vi "Control iteration 0.vi"(4 "Angle theta [degrees]":dbl, 6 "Number of steps":dbl, 7 "Sweep plane & fixed axis":string, 9 "Current iteration":i32, 10 "Magnetic field strength [µT]":dbl, 11 "Octant":string) -> (0 "Magnetic field z [µT]":dbl, 1 "Magnetic field y [µT]":dbl, 2 "Magnetic field x [µT]":dbl, 3 "Current angle":dbl, 5 "Output instructions iteration 0":string)   [LabVIEW 2018]
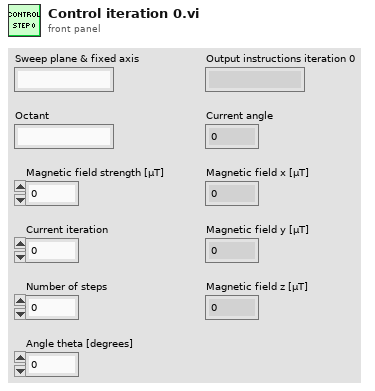
[diagram p1: front panel]
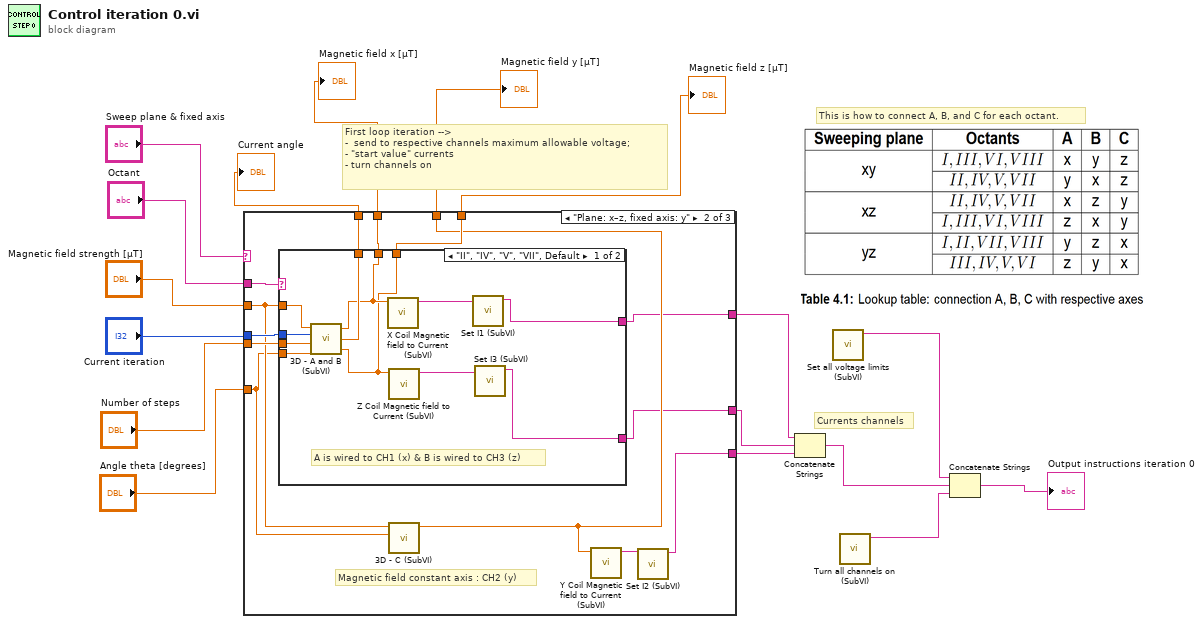
[diagram p0: block diagram]
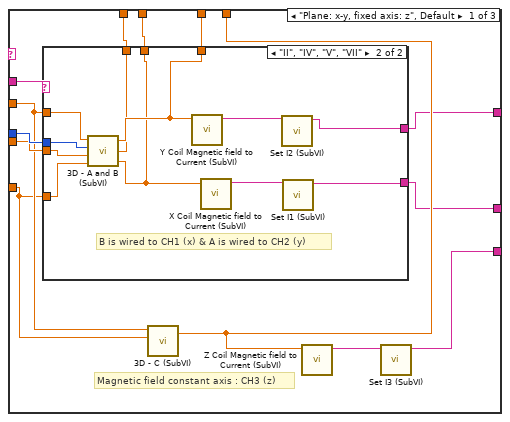
[diagram p2: hidden frame]
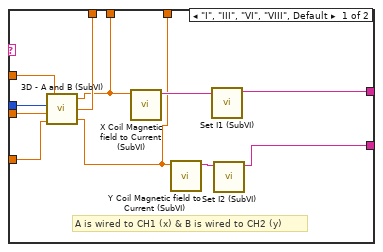
[diagram p3: hidden frame]
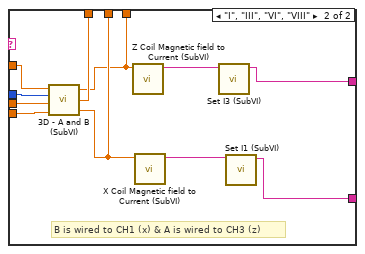
[diagram p4: hidden frame]
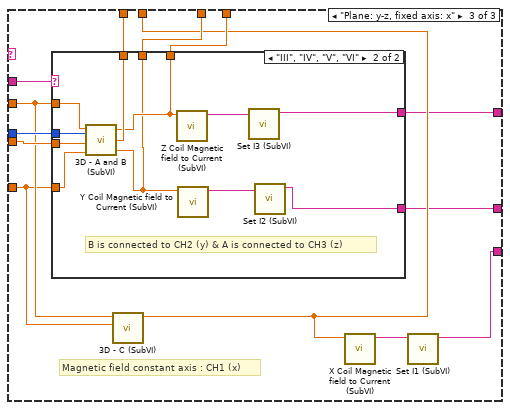
[diagram p5: hidden frame]
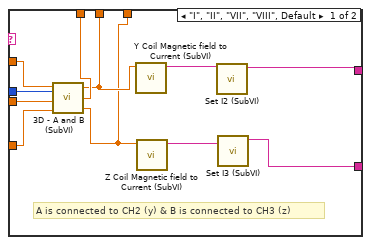
[diagram p6: hidden frame]
diagram:
  # "This is how to connect A, B, and C for each octant."
  # "Currents channels"
  # "First loop iteration -->\n-  send to respective channels maximum allowable voltage;\n- \"start value\" currents\n- turn channels on"
  n1 = case shown="\"Plane: x–z, fixed axis: y\"" "Sweep plane & fixed axis" {
    tunnel: "Octant" -> [w30 w65 w100]
    tunnel: "Magnetic field strength [µT]" -> [w24 w59 w94]
    tunnel: "Current iteration" -> [w29 w63 w99]
    tunnel: "Number of steps" -> [w28 w64 w98]
    tunnel: "Angle theta [degrees]" -> [w23 w58 w93]
    tunnel: [w27 w62 w97] -> w13
    tunnel: [w26 w61 w92] -> w1
    tunnel: [w25 w57 w95] -> w2
    tunnel: [w22 w60 w96] -> w3
    tunnel: [w18 w53 w88] -> w14
    tunnel: [w21 w56 w91] -> w15
    tunnel: [w20 w55 w90] -> w16
    frame "Plane: x-y, fixed axis: z", Default {
      # "Magnetic field constant axis : CH3 (z)"
      n2 = case shown="\"II\", \"IV\", \"V\", \"VII\"" w30 {
        tunnel: w24 -> [w41 w52]
        tunnel: w29 -> [w40 w51]
        tunnel: w28 -> [w39 w50]
        tunnel: w23 -> [w38 w49]
        tunnel: [w37 w42] -> w27
        tunnel: [w34 w46] -> w20
        tunnel: [w33 w44] -> w21
        tunnel: [w32 w43] -> w26
        tunnel: [w31 w48] -> w25
        frame "I", "III", "VI", "VIII", Default {
          # "A is wired to CH1 (x) & B is wired to CH2 (y)"
          n3 = call "3D - A and B (SubVI).vi"("Angle theta [degrees]"=w38, "Total steps"=w39, "Current step"=w40, "Magnitude"=w41) -> ("B_B"=w31:dbl, "Current angle"=w37:dbl, "B_A"=w32:dbl)
          n4 = call "X Coil Magnetic field to Current (SubVI).vi"("Magnetic field [µT]"=w32) -> ("Current X"=w36:string)  [unwired: 10 in]
          n5 = call "Y Coil Magnetic field to Current (SubVI).vi"("Magnetic field [µT]"=w31) -> ("Current Y"=w35:string)  [unwired: 10 in]
          n6 = call "Set I1 (SubVI).vi"("Current X"=w36) -> ("String instruction"=w34:string)  [unwired: 10 in]
          n7 = call "Set I2 (SubVI).vi"("Current Y"=w35) -> ("String"=w33:string)  [unwired: 10 in]
        }
        frame "II", "IV", "V", "VII" {
          # "B is wired to CH1 (x) & A is wired to CH2 (y)"
          n8 = call "3D - A and B (SubVI).vi"("Angle theta [degrees]"=w49, "Total steps"=w50, "Current step"=w51, "Magnitude"=w52) -> ("B_B"=w43:dbl, "Current angle"=w42:dbl, "B_A"=w48:dbl)
          n9 = call "Y Coil Magnetic field to Current (SubVI).vi"("Magnetic field [µT]"=w48) -> ("Current Y"=w47:string)  [unwired: 10 in]
          n10 = call "X Coil Magnetic field to Current (SubVI).vi"("Magnetic field [µT]"=w43) -> ("Current X"=w45:string)  [unwired: 10 in]
          n11 = call "Set I2 (SubVI).vi"("Current Y"=w47) -> ("String"=w46:string)  [unwired: 10 in]
          n12 = call "Set I1 (SubVI).vi"("Current X"=w45) -> ("String instruction"=w44:string)  [unwired: 10 in]
        }
      }
      n13 = call "3D - C (SubVI).vi"("Angle theta"=w23, "Magnitude"=w24) -> ("B_C"=w22:dbl)  [unwired: 9 in]
      n14 = call "Z Coil Magnetic field to Current (SubVI).vi"("Magnetic field [µT]"=w22) -> ("Current Z"=w19:string)  [unwired: 10 in]
      n15 = call "Set I3 (SubVI).vi"("Current Z"=w19) -> ("String"=w18:string)  [unwired: 10 in]
    }
    frame "Plane: x–z, fixed axis: y" {
      # "Magnetic field constant axis : CH2 (y)"
      n16 = case shown="\"II\", \"IV\", \"V\", \"VII\", Default" w65 {
        tunnel: [w68 w81] -> w56
        tunnel: [w70 w82] -> w55
        tunnel: w64 -> [w74 w87]
        tunnel: w63 -> [w75 w86]
        tunnel: w59 -> [w76 w85]
        tunnel: w58 -> [w73 w84]
        tunnel: [w72 w79] -> w62
        tunnel: [w67 w78] -> w61
        tunnel: [w66 w77] -> w60
        frame "II", "IV", "V", "VII", Default {
          # "A is wired to CH1 (x) & B is wired to CH3 (z)"
          n17 = call "3D - A and B (SubVI).vi"("Angle theta [degrees]"=w73, "Total steps"=w74, "Current step"=w75, "Magnitude"=w76) -> ("B_B"=w66:dbl, "Current angle"=w72:dbl, "B_A"=w67:dbl)
          n18 = call "X Coil Magnetic field to Current (SubVI).vi"("Magnetic field [µT]"=w67) -> ("Current X"=w71:string)  [unwired: 10 in]
          n19 = call "Z Coil Magnetic field to Current (SubVI).vi"("Magnetic field [µT]"=w66) -> ("Current Z"=w69:string)  [unwired: 10 in]
          n20 = call "Set I1 (SubVI).vi"("Current X"=w71) -> ("String instruction"=w70:string)  [unwired: 10 in]
          n21 = call "Set I3 (SubVI).vi"("Current Z"=w69) -> ("String"=w68:string)  [unwired: 10 in]
        }
        frame "I", "III", "VI", "VIII" {
          # "B is wired to CH1 (x) & A is wired to CH3 (z)"
          n22 = call "3D - A and B (SubVI).vi"("Angle theta [degrees]"=w84, "Total steps"=w87, "Current step"=w86, "Magnitude"=w85) -> ("B_B"=w78:dbl, "Current angle"=w79:dbl, "B_A"=w77:dbl)
          n23 = call "Z Coil Magnetic field to Current (SubVI).vi"("Magnetic field [µT]"=w77) -> ("Current Z"=w83:string)  [unwired: 10 in]
          n24 = call "X Coil Magnetic field to Current (SubVI).vi"("Magnetic field [µT]"=w78) -> ("Current X"=w80:string)  [unwired: 10 in]
          n25 = call "Set I3 (SubVI).vi"("Current Z"=w83) -> ("String"=w82:string)  [unwired: 10 in]
          n26 = call "Set I1 (SubVI).vi"("Current X"=w80) -> ("String instruction"=w81:string)  [unwired: 10 in]
        }
      }
      n27 = call "3D - C (SubVI).vi"("Angle theta"=w58, "Magnitude"=w59) -> ("B_C"=w57:dbl)  [unwired: 9 in]
      n28 = call "Y Coil Magnetic field to Current (SubVI).vi"("Magnetic field [µT]"=w57) -> ("Current Y"=w54:string)  [unwired: 10 in]
      n29 = call "Set I2 (SubVI).vi"("Current Y"=w54) -> ("String"=w53:string)  [unwired: 10 in]
    }
    frame "Plane: y-z, fixed axis: x" {
      # "Magnetic field constant axis : CH1 (x)"
      n30 = case shown="\"III\", \"IV\", \"V\", \"VI\"" w100 {
        tunnel: [w103 w112] -> w90
        tunnel: [w101 w114] -> w91
        tunnel: w94 -> [w111 w122]
        tunnel: w99 -> [w110 w121]
        tunnel: w98 -> [w109 w120]
        tunnel: w93 -> [w108 w119]
        tunnel: [w107 w118] -> w97
        tunnel: [w105 w117] -> w96
        tunnel: [w106 w116] -> w95
        frame "I", "II", "VII", "VIII", Default {
          # "A is connected to CH2 (y) & B is connected to CH3 (z)"
          n31 = call "3D - A and B (SubVI).vi"("Angle theta [degrees]"=w108, "Total steps"=w109, "Current step"=w110, "Magnitude"=w111) -> ("B_B"=w105:dbl, "Current angle"=w107:dbl, "B_A"=w106:dbl)
          n32 = call "Y Coil Magnetic field to Current (SubVI).vi"("Magnetic field [µT]"=w106) -> ("Current Y"=w104:string)  [unwired: 10 in]
          n33 = call "Z Coil Magnetic field to Current (SubVI).vi"("Magnetic field [µT]"=w105) -> ("Current Z"=w102:string)  [unwired: 10 in]
          n34 = call "Set I2 (SubVI).vi"("Current Y"=w104) -> ("String"=w103:string)  [unwired: 10 in]
          n35 = call "Set I3 (SubVI).vi"("Current Z"=w102) -> ("String"=w101:string)  [unwired: 10 in]
        }
        frame "III", "IV", "V", "VI" {
          # "B is connected to CH2 (y) & A is connected to CH3 (z)"
          n36 = call "3D - A and B (SubVI).vi"("Angle theta [degrees]"=w119, "Total steps"=w120, "Current step"=w121, "Magnitude"=w122) -> ("B_B"=w116:dbl, "Current angle"=w118:dbl, "B_A"=w117:dbl)
          n37 = call "Z Coil Magnetic field to Current (SubVI).vi"("Magnetic field [µT]"=w117) -> ("Current Z"=w113:string)  [unwired: 10 in]
          n38 = call "Y Coil Magnetic field to Current (SubVI).vi"("Magnetic field [µT]"=w116) -> ("Current Y"=w115:string)  [unwired: 10 in]
          n39 = call "Set I3 (SubVI).vi"("Current Z"=w113) -> ("String"=w112:string)  [unwired: 10 in]
          n40 = call "Set I2 (SubVI).vi"("Current Y"=w115) -> ("String"=w114:string)  [unwired: 10 in]
        }
      }
      n41 = call "3D - C (SubVI).vi"("Angle theta"=w93, "Magnitude"=w94) -> ("B_C"=w92:dbl)  [unwired: 9 in]
      n42 = call "X Coil Magnetic field to Current (SubVI).vi"("Magnetic field [µT]"=w92) -> ("Current X"=w89:string)  [unwired: 10 in]
      n43 = call "Set I1 (SubVI).vi"("Current X"=w89) -> ("String instruction"=w88:string)  [unwired: 10 in]
    }
  }
  "Magnetic field y [µT]" <- w2
  "Magnetic field z [µT]" <- w3
  "Magnetic field x [µT]" <- w1
  "Current angle" <- w13
  n44 = Concatenate Strings(w16, w15, w14) -> (w17:string)
  n45 = call "Set all voltage limits (SubVI).vi"() -> ("String"=w7:string)  [unwired: 11 in]
  n46 = call "Turn all channels on (SubVI).vi"() -> ("String"=w5:string)  [unwired: 11 in]
  n47 = Concatenate Strings(w7, w17, w5) -> (→"Output instructions iteration 0":string)
